vi "New Verify as Parameterized.vi"(11 "LUnit Test Case In":refnum<class "Test Case.lvclass">) -> (0 "error out":errorcluster, 3 "LUnit Test Case Out":refnum<class "Test Case.lvclass">)   [LabVIEW 2020, in "LUnit.Extension.lvlib"]
uses:
  LUnit.Extension.lvlib
  <vilib>/Astemes/LUnit/Test Case.lvclass
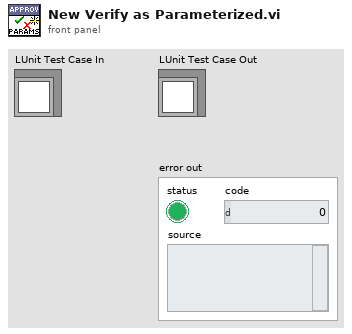
[diagram p1: front panel]
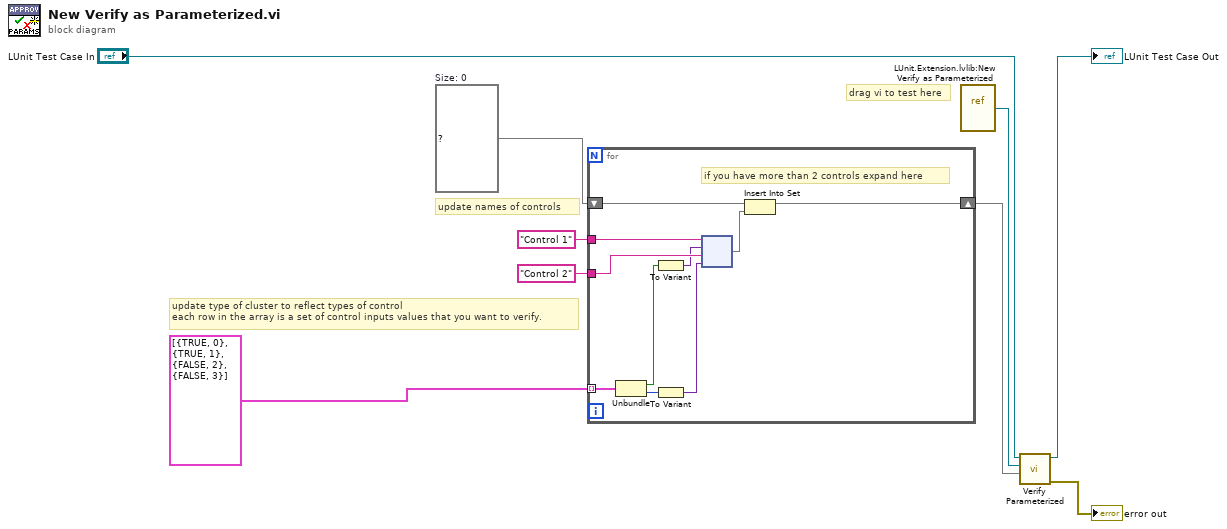
[diagram p0: block diagram]
diagram:
  w4 = set{map{string, variant}} {}  # Size: 0
  # "update type of cluster to reflect types of control\neach row in the array is a set of control inputs values that you want to verify."
  # "update names of controls"
  # "drag vi to test here"
  n1 = for {
    tunnel: "Control 1" -> [w19]
    tunnel: cluster{bool, i32}[] [{TRUE, 0}, {TRUE, 1}, {FALSE, 2}, {FALSE, 3}] -> [w17] mode=indexing
    tunnel: "Control 2" -> [w18]
    shift-right: [w11] -> w3
    shift-left: w4 -> [w10]
    # "if you have more than 2 controls expand here"
    n2 = Unbundle(w17) -> (w16:bool, w15:i32)
    n3 = To Variant(anything=w16) -> (Variant=w13:variant)
    n4 = To Variant(anything=w15) -> (Variant=w12:variant)
    n5 = node(w19, w13, w18, w12) -> (w14:map{string, variant})
    n6 = Insert Into Set(10:w14, 11:w10) -> (3:w11:set{map{string, variant}})  [unwired: 1 out]
  }
  n7 = vi-ref "LUnit.Extension.lvlib:New Verify as Parameterized.vi"() -> (w8:refnum<vi>)
  n8 = call "Verify Parameterized.vi"("Set of ctl label -> value var"=w3, "VI in"=w8, "LUnit Test Case In"="LUnit Test Case In") -> ("error out"=→"error out":errorcluster, "LUnit Test Case Out"=→"LUnit Test Case Out":refnum<class "Test Case.lvclass">)  [unwired: 7 in]
